vi "Configure Bus Source (AUDIO - Frame).vi"(0 "VISA resource name":refnum<visa-resource-name>, 1 "Word Select Polarity (0: Normal)":u16(ring) items=["Normal", "Invert"], 5 "BUS Number (9: Bus 1)":u16(ring)=9 items=["Bus 1"=9, "Bus 2"=10, "Bus 3"=11, "Bus 4"=12], 7 "Framesync Source (0: Channel 1)":u16(ring) items=["Channel 1"=0, "Channel 2"=1, "Channel 3"=2, "Channel 4"=3, "Digital Channel 0"=14, "Digital Channel 1"=15, "Digital Channel 2"=16, "Digital Channel 3"=17, "Digital Channel 4"=18, "Digital Channel 5"=19, "Digital Channel 6"=20, "Digital Channel 7"=21, "Digital Channel 8"=22, "Digital Channel 9"=23, "Digital Channel 10"=24, "Digital Channel 11"=25, "Digital Channel 12"=26, "Digital Channel 13"=27, "Digital Channel 14"=28, "Digital Channel 15"=29], 9 "Framesync Polarity (0: Fall)":u16(ring) items=["Fall", "Rise"], 11 "error in (no error)":errorcluster, 12 "Word Select Source (0: Channel 1)":u16(ring) items=["Channel 1"=0, "Channel 2"=1, "Channel 3"=2, "Channel 4"=3, "Digital Channel 0"=14, "Digital Channel 1"=15, "Digital Channel 2"=16, "Digital Channel 3"=17, "Digital Channel 4"=18, "Digital Channel 5"=19, "Digital Channel 6"=20, "Digital Channel 7"=21, "Digital Channel 8"=22, "Digital Channel 9"=23, "Digital Channel 10"=24, "Digital Channel 11"=25, "Digital Channel 12"=26, "Digital Channel 13"=27, "Digital Channel 14"=28, "Digital Channel 15"=29]) -> (4 "VISA resource name out":refnum<visa-resource-name>, 15 "error out":errorcluster)   [LabVIEW 2010, in "Tektronix DPO MSO 2000 4000 Series.lvlib"]
doc: "This VI sets the frame sync settings for the AUDIO bus.\n\n<B>Note:</B> This VI is only valid if you have installed the AUDIO application module."
uses:
  <instrlib>/Tektronix DPO MSO 2000 4000 Series/Tektronix DPO MSO 2000 4000 Series.lvlib
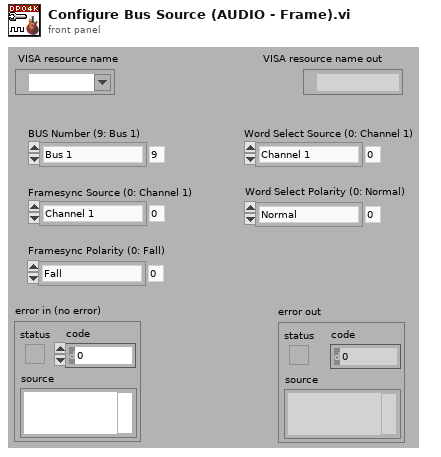
[diagram p1: front panel]
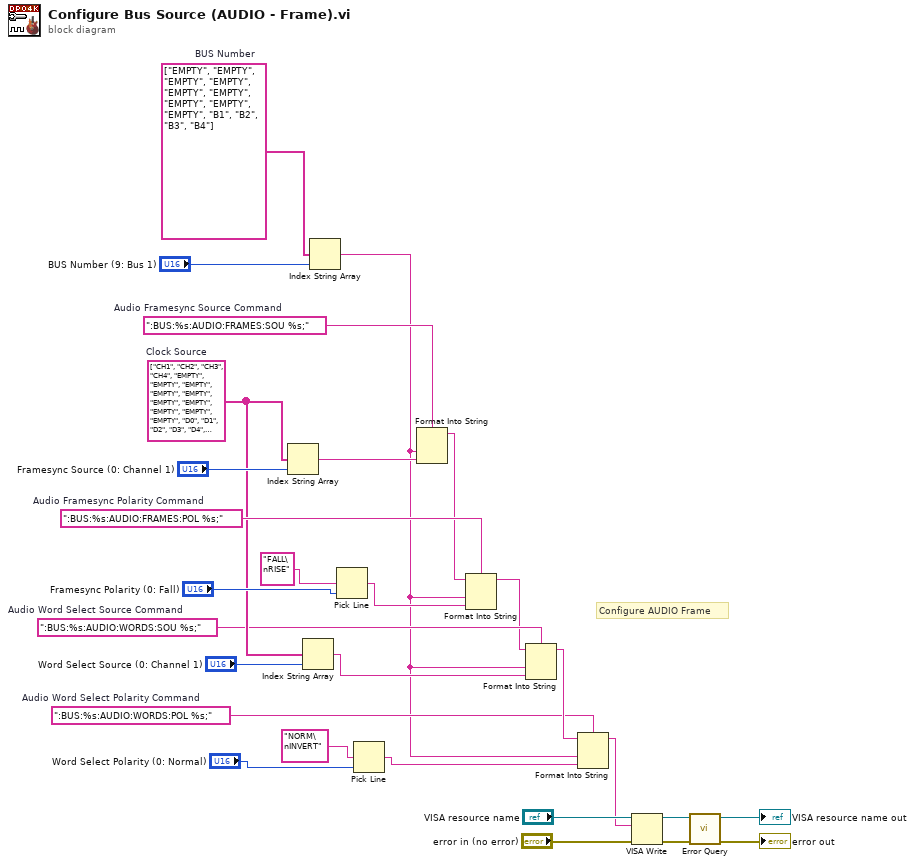
[diagram p0: block diagram]
diagram:
  w4 = ":BUS:%s:AUDIO:WORDS:POL %s;"  # Audio Word Select Polarity Command
  w10 = ":BUS:%s:AUDIO:WORDS:SOU %s;"  # Audio Word Select Source Command
  w21 = ":BUS:%s:AUDIO:FRAMES:POL %s;"  # Audio Framesync Polarity Command
  w12 = string[] ["CH1", "CH2", "CH3", "CH4", "EMPTY", "EMPTY", "EMPTY", "EMPTY", "EMPTY", "EMPTY", "EMPTY", "EMPTY", "EMPTY", "EMPTY", "D0", "D1", "D2", "D3", "D4", "D5", "D6", "D7", "D8", "D9", "D10", "D11", "D12", "D13", "D14", "D15"]  # Clock Source
  w26 = ":BUS:%s:AUDIO:FRAMES:SOU %s;"  # Audio Framesync Source Command
  w28 = string[] ["EMPTY", "EMPTY", "EMPTY", "EMPTY", "EMPTY", "EMPTY", "EMPTY", "EMPTY", "EMPTY", "B1", "B2", "B3", "B4"]  # BUS Number
  # "Configure AUDIO Frame"
  n1 = Index String Array(1:"Framesync Source (0: Channel 1)", 2:w12) -> (0:w24:string)  [unwired: 1 in]
  n2 = Index String Array(1:"Word Select Source (0: Channel 1)", 2:w12) -> (0:w9:string)  [unwired: 1 in]
  n3 = Index String Array(1:"BUS Number (9: Bus 1)", 2:w28) -> (0:w3:string)  [unwired: 1 in]
  n4 = Pick Line(multi-line string="FALL\nRISE", line index="Framesync Polarity (0: Fall)") -> (output string=w20:string)  [unwired: 1 in]
  n5 = Pick Line(multi-line string="NORM\nINVERT", line index="Word Select Polarity (0: Normal)") -> (output string=w2:string)  [unwired: 1 in]
  n6 = Format Into String(format string=w26, w3, w24) -> (resulting string=w19:string)  [unwired: 2 in, 1 out]
  n7 = Format Into String(format string=w21, initial string=w19, w3, w20) -> (resulting string=w8:string)  [unwired: 1 in, 1 out]
  n8 = Format Into String(format string=w10, initial string=w8, w3, w9) -> (resulting string=w5:string)  [unwired: 1 in, 1 out]
  n9 = Format Into String(format string=w4, initial string=w5, w3, w2) -> (resulting string=w1:string)  [unwired: 1 in, 1 out]
  n10 = VISA Write(VISA resource name="VISA resource name", write buffer=w1, error in (no error)="error in (no error)") -> (VISA resource name out=w16:refnum<visa-resource-name>, error out=w15:errorcluster)  [unwired: 1 out]
  n11 = call <instrlib>:"Error Query.vi"("error in (no error)"=w15, "VISA resource name"=w16) -> ("error out"=→"error out":errorcluster, "VISA resource name out"=→"VISA resource name out":refnum<visa-resource-name>)  [unwired: 6 in, 2 out]
